vi "Uniquify_Label.vi"(8 "error in (no error)":errorcluster, 10 "names":string[](array[string]), 11 "absFolder in":refnum<class "absFolder.lvclass">) -> (0 "error out":errorcluster, 2 "names":string, 3 "absFolder out":refnum<class "absFolder.lvclass">)   [LabVIEW 2020, in "absFolder.lvclass"]
uses:
  <vilib>/AppBuilder/IB_Classes/Destination/absFolder/absFolder.lvclass
  <vilib>/AppBuilder/IB_Classes/Destination/absFolder/absFolder.lvclass/absFolder.ctl
  <resource>/Framework/Providers/Builds/Installer/CDK_GLOBAL_STRINGS.vi
  <vilib>/AppBuilder/IB_Classes/Destination/IB_Destination.lvclass
  e:/builds/penguin/labview/branches/2020/dev/dist/vi.lib/AppBuilder/IB_Classes/Destination/IB_Destination.lvclass
  e:/builds/penguin/labview/branches/2020/dev/dist/vi.lib/AppBuilder/IB_Classes/Destination/absFolder/absFolder.lvclass
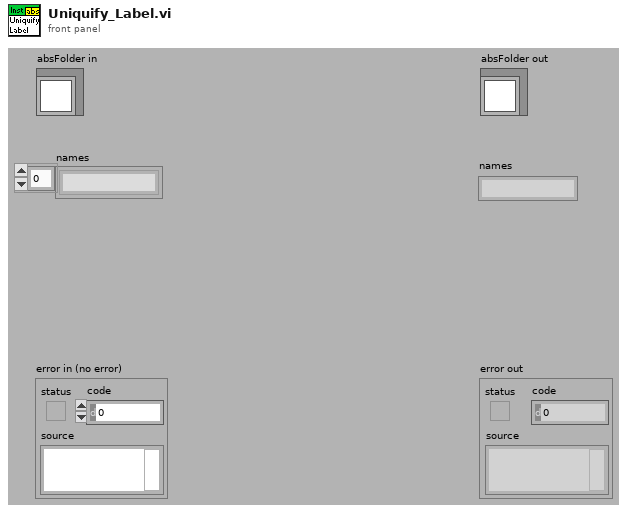
[diagram p1: front panel]
types:
  T1 = typedef "IB_Destination.ctl" = cluster{"name":string, "unlock":bool, "parentTag":string, "destTag":string, "eng_installPath":string}
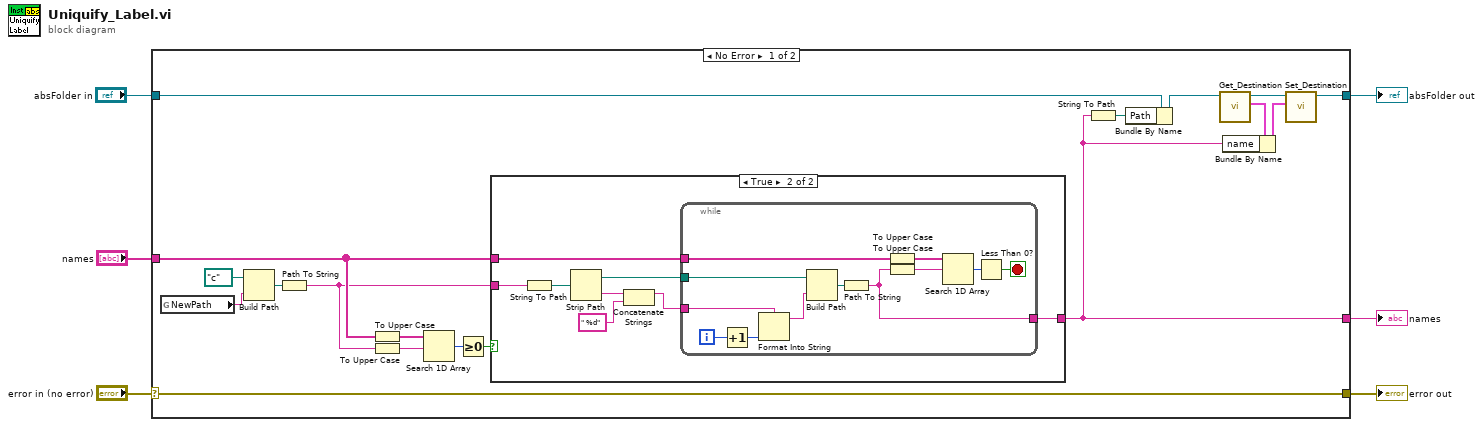
[diagram p0: block diagram]
diagram:
  n1 = case shown="No Error" "error in (no error)" {
    selector: "error in (no error)" -> [w24 w47]
    tunnel: [w24 w47] -> w4
    tunnel: "names" -> [w19 _]
    tunnel: [w9 _] -> w3
    tunnel: "absFolder in" -> [w14 w46]
    tunnel: [w7 w46] -> w1
    frame No Error {
      n2 = global read "CDK_GLOBAL_STRINGS.vi" "NewPath"() -> (w17:string)
      n3 = Build Path(base path=path "c:/", name or relative path=w17) -> (appended path=w18:path)
      n4 = Path To String(path=w18) -> (string=w15:string)
      n5 = To Upper Case(1:w19) -> (0:w21:string[])
      n6 = To Upper Case(1:w15) -> (0:w20:string)
      n7 = Search 1D Array(1D array=w21, element=w20) -> (index of element=w23:i32)  [unwired: 1 out]
      n8 = Greater Or Equal To 0?(x=w23) -> (x >= 0?=w22:bool)
      n9 = case shown="True" w22 {
        tunnel: w19 -> [_ w33]
        tunnel: w15 -> [w25 w30]
        tunnel: [w25 w31] -> w9
        frame False {
        }
        frame True {
          n10 = String To Path(string=w30) -> (path=w29:path)
          n11 = Strip Path(path=w29) -> (stripped path=w26:path, name=w28:string)
          n12 = Concatenate Strings(w28, " %d" ("string")) -> (w27:string)
          n13 = while {
            tunnel: w33 -> [w42]
            tunnel: [w34] -> w31
            tunnel: w27 -> [w38]
            tunnel: w26 -> [w36]
            i -> [w39]
            stop <- w44 stop-if-true
            n14 = Increment(x=w39) -> (x+1=w40:i32)
            n15 = Format Into String(format string=w38, w40) -> (resulting string=w35:string)  [unwired: 2 in, 1 out]
            n16 = Build Path(base path=w36, name or relative path=w35) -> (appended path=w37:path)
            n17 = Path To String(path=w37) -> (string=w34:string)
            n18 = To Upper Case(1:w42) -> (0:w43:string[])
            n19 = To Upper Case(1:w34) -> (0:w41:string)
            n20 = Search 1D Array(1D array=w43, element=w41) -> (index of element=w45:i32)  [unwired: 1 out]
            n21 = Less Than 0?(x=w45) -> (x < 0?=w44:bool)
          }
        }
      }
      n22 = String To Path(string=w9) -> (path=w13:path)
      n23 = Bundle By Name(cluster=w14, "Path"=w13) -> (w8:refnum<class "absFolder.lvclass">)
      n24 = call <vilib>:"Get_Destination.vi"("IB_Destination in"=w8) -> ("data"=w11:T1, "IB_Destination out"=w12:refnum<class "absFolder.lvclass">)  [unwired: 1 in, 8 out]
      n25 = Bundle By Name(cluster=w11, "name"=w9) -> (w10:T1)
      n26 = call <vilib>:"Set_Destination.vi"("data"=w10, "IB_Destination in"=w12) -> ("IB_Destination out"=w7:refnum<class "absFolder.lvclass">)  [unwired: 1 in, 8 out]
    }
    frame Error {
    }
  }
  "error out" <- w4
  "absFolder out" <- w1
  "names" <- w3
